vi "FF_AnkleTrajAdv2.vi"(6 "Init":bool, 7 "dt":dbl=0.01 format="%0.2f", 8 "error in (no error)":errorcluster, 9 "AnkleVelocity":dbl[](array[numeric]), 10 "AnkleInGCS":dbl[](array[numeric]), 11 "Force Field Controller in":refnum<class "ForceField.lvclass">) -> (0 "error out":errorcluster, 1 "ClosestPoint":dbl[](array[numeric]), 2 "ForceXYZ":dbl[](array[numeric]), 3 "Force Field Controller out":refnum<class "ForceField.lvclass">, 4 "UpdateTrajPrev":bool, 5 "ForceNTD":dbl[](array[numeric]))   [LabVIEW 2015, in "ForceField.lvclass"]
uses:
  ForceField.lvclass
  ForceField.lvclass/ForceField.ctl
  TypeDef/TND.ctl
  <vilib>/ptbypt/NI_PtbyPt.lvlib
panel:
  out "ToeOffIdx":i32
  in  "3D":bool
  in  "Adv?":bool=TRUE
  out "weightPrev":dbl
  out "ClosePt 2":dbl[](array[numeric])
  in  "HalfWindow 2":i32=35
  in  "dXmin":dbl=0.2 format="%#_13g"
  in  "HalfWindow 1":i32=35
  out "ClosePt 1":dbl[](array[numeric])
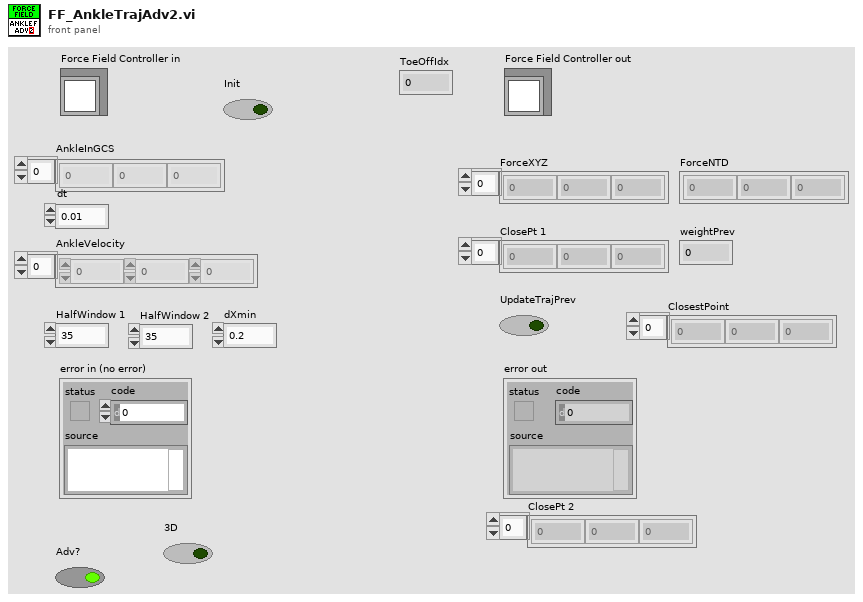
[diagram p1: front panel]
types:
  T1 = typedef "ForceField.lvclass/TND.ctl" = cluster{"Vt":dbl[], "Vn":dbl[], "Dmin":dbl}
  T2 = typedef "ForceField.lvclass/AnkleTrajPt.ctl" = cluster{"P1":dbl[], "P2":dbl[], "P1-P2":dbl[], "(P1-P2)^2":dbl}
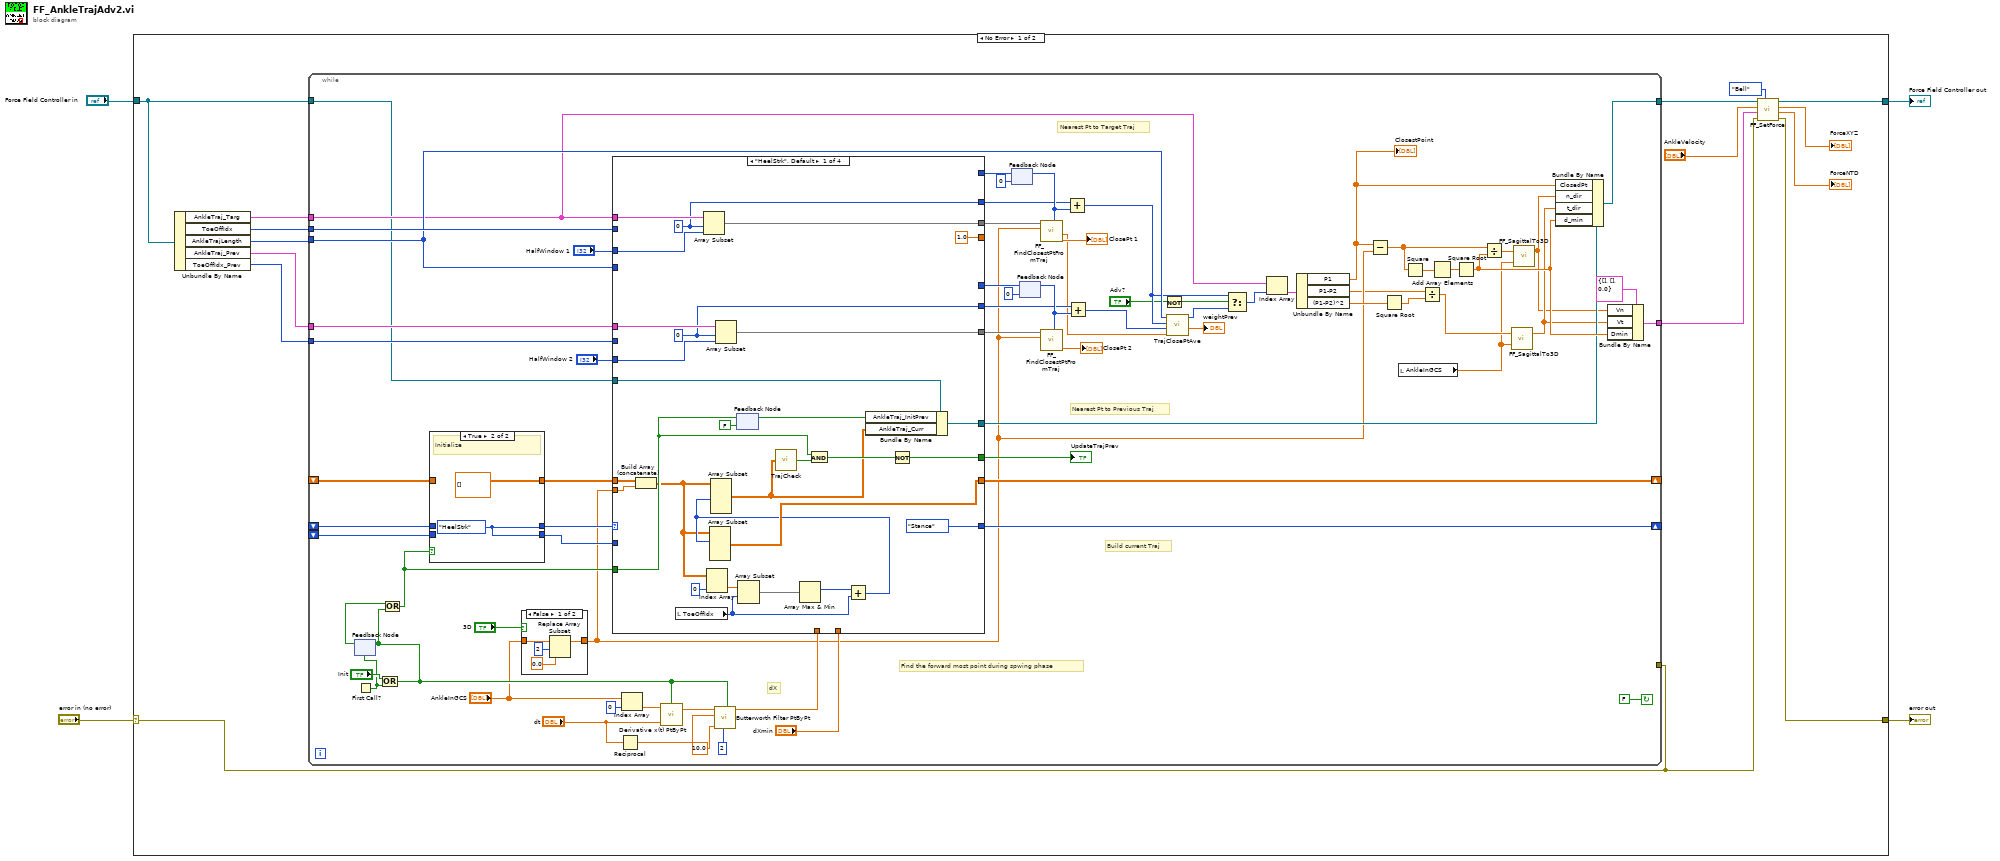
[diagram p0: block diagram]
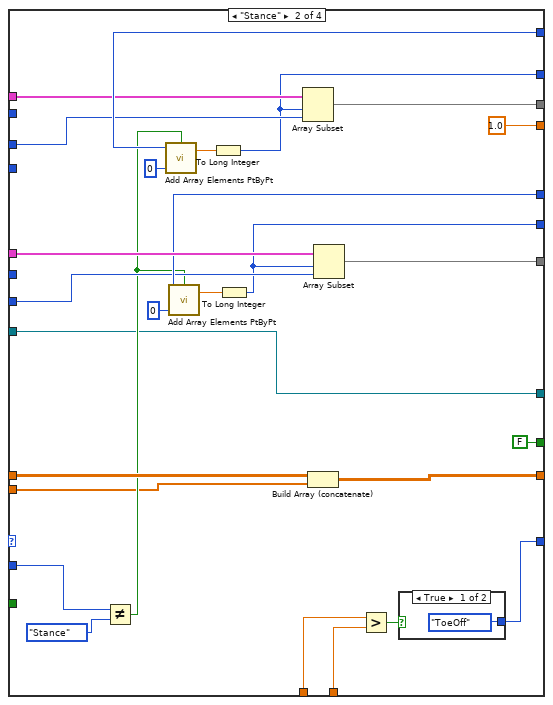
[diagram p3: hidden frame]
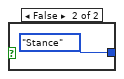
[diagram p4: hidden frame]
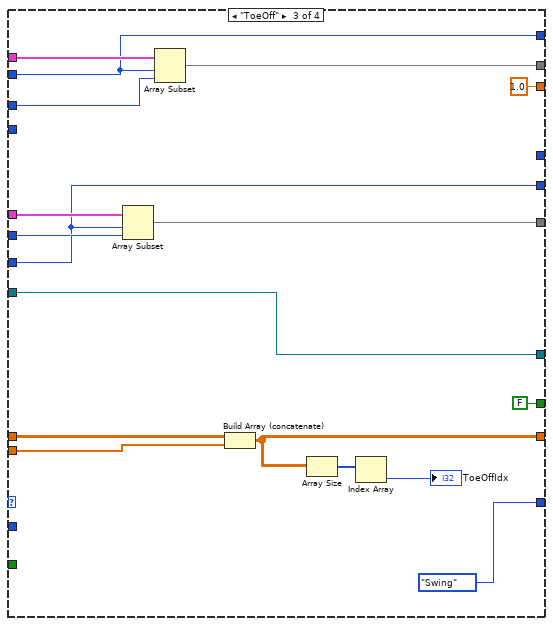
[diagram p5: hidden frame]
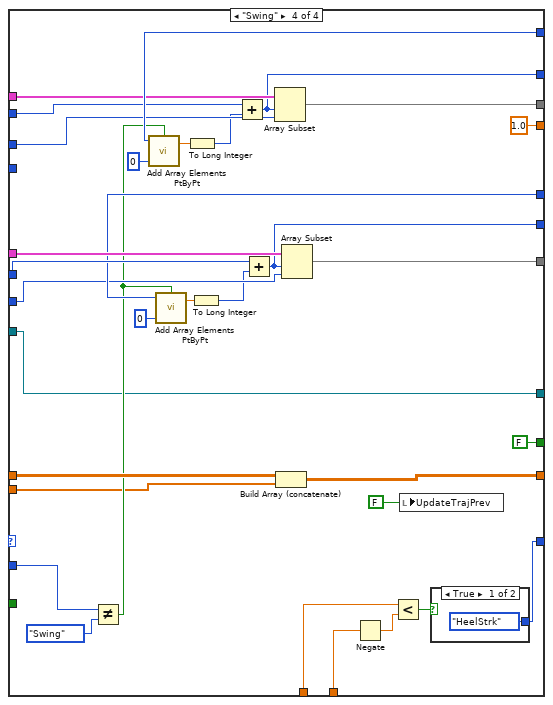
[diagram p6: hidden frame]
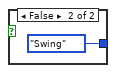
[diagram p7: hidden frame]
diagram:
  n1 = case shown="No Error" "error in (no error)" {
    selector: "error in (no error)" -> [w5 w214]
    tunnel: [w17 w214] -> w3
    tunnel: [w18 w213] -> w1
    tunnel: "Force Field Controller in" -> [w19 w213]
    frame No Error {
      n2 = Unbundle By Name(w19) -> ("AnkleTraj_Targ"=w15:T2[], "ToeOffIdx"=w14:i32, "AnkleTrajLength"=w13:i32, "AnkleTraj_Prev"=w7:T2[], "ToeOffIdx_Prev"=w6:i32)
      n3 = while {
        tunnel: w15 -> [w73]
        tunnel: w14 -> [w84]
        tunnel: w19 -> [w41]
        tunnel: [w92] -> w16
        shift-right: [w87] -> _
        shift-left: _ -> [w79]
        shift-left: _ -> [w77]
        shift-right: [w86] -> _
        shift-left: _ -> [w81]
        tunnel: w13 -> [w82]
        tunnel: w7 -> [w85]
        tunnel: w6 -> [w83]
        tunnel: [w64] -> w12
        tunnel: w5 -> [_]
        stop <- FALSE continue-if-true
        # "dX"
        # "Find the forward most point during spwing phase"
        # "Nearest Pt to Previous Traj"
        # "Build current Traj"
        # "Nearest Pt to Target Traj"
        n4 = First Call?() -> (First Call?: T/F=w74:bool)
        n5 = feedback #1(w74) -> (w75:bool)
        n6 = Or(x="Init", y=w74) -> (x .or. y?=w36:bool)
        n7 = feedback-in #1(w36) -> ()
        n8 = Or(x=w75, y=w36) -> (x .or. y?=w63:bool)
        n9 = case shown="True" w63 {
          tunnel: w81 -> [w210 _]
          tunnel: [w210 dbl[][] []] -> w80
          tunnel: w79 -> [w209 _]
          tunnel: [w209 w211] -> w78
          tunnel: w77 -> [w208 _]
          tunnel: [w208 w211] -> w76
          frame False {
          }
          frame True {
            w211 = enum16{"HeelStrk", "Stance", "ToeOff", "Swing"}."HeelStrk"
            # "Initialize"
          }
        }
        n10 = case shown="False" "3D" {
          tunnel: "AnkleInGCS" -> [w96 w97]
          tunnel: [w95 w97] -> w27
          frame False {
            n11 = Replace Array Subset(array=w96, new element=0.0 ("new element/subarray"), index=2) -> (w95:dbl[])
          }
          frame True {
          }
        }
        n12 = Reciprocal(x="dt") -> (1/x=w34:dbl)
        n13 = Index Array(array="AnkleInGCS", index=0) -> (element=w28:dbl)
        n14 = call <vilib>:"Derivative x(t) PtByPt.vi"("initialize"=w36, "dt"="dt", "x"=w28) -> ("dx/dt"=w38:dbl)  [unwired: 1 in, 1 out]
        n15 = call <vilib>:"Butterworth Filter PtByPt.vi"("initialize"=w36, "order"=2, "low cutoff freq: fl"=10.0, "sampling freq: fs"=w34, "x"=w38) -> ("Filtered x"=w29:dbl)  [unwired: 4 in, 1 out]
        n16 = feedback #2(0 ("IndexOfClosePt")) -> (w61:i32)
        n17 = feedback #3(0 ("IndexOfClosePt")) -> (w55:i32)
        n18 = case shown="\"HeelStrk\", Default" w78 {
          tunnel: w73 -> [w123 w145 w167 w191]
          tunnel: "HalfWindow 1" -> [w124 w152 w170 w204]
          tunnel: [w126 w149 w172 w201] -> w59
          tunnel: [enum16{"HeelStrk", "Stance", "ToeOff", "Swing"}."Stance" w148 enum16{"HeelStrk", "Stance", "ToeOff", "Swing"}."Swing" w199] -> w87
          tunnel: w61 -> [_ w153 _ w205]
          tunnel: w29 -> [_ w147 _ w198]
          tunnel: w76 -> [_ w144 _ w197]
          tunnel: [1.0 1.0 1.0 1.0] -> _
          tunnel: "dXmin" -> [_ w142 _ w194]
          tunnel: w27 -> [w112 w128 w160 w174]
          tunnel: [w105 w141 w158 w192] -> w86
          tunnel: w80 -> [w107 w140 w168 w193]
          tunnel: w82 -> [_ _ _ _]
          tunnel: w85 -> [w121 w138 w166 w186]
          tunnel: "HalfWindow 2" -> [w120 w135 w164 w183]
          tunnel: [w119 w136 w165 w182] -> w54
          tunnel: w84 -> [_ _ w163 w189]
          tunnel: w55 -> [_ w137 _ w184]
          tunnel: w83 -> [_ _ w162 w185]
          tunnel: [w117 w130 w162 w180] -> w51
          tunnel: [w118 w131 w163 w179] -> w49
          tunnel: w63 -> [w108 _ _ _]
          tunnel: w41 -> [w115 w129 w161 w175]
          tunnel: [w113 w129 w161 w175] -> w40
          tunnel: [w110 FALSE FALSE FALSE] -> w30
          frame "HeelStrk", Default {
            w117 = 0 ("index")
            w118 = 0 ("index")
            n19 = Build Array (concatenate)(w107, w112) -> (w103:dbl[][])
            n20 = local read "ToeOffIdx"() -> (w99:i32)
            n21 = Array Subset(array=w123, index=w118, length=w124) -> (w126:T2[])
            n22 = Index Array(array=w103, index (col)=0 ("disabled index (col)")) -> (element=w101:dbl[])  [unwired: 1 in]
            n23 = Array Subset(array=w121, index=w117, length=w120) -> (w119:T2[])
            n24 = feedback-in #4(w108) -> ()
            n25 = feedback #4(FALSE) -> (w114:bool)
            n26 = Array Subset(array=w101, index=w99) -> (w100:dbl[])  [unwired: 1 in]
            n27 = Array Max & Min(array=w100) -> (max index (indices)=w98:i32)  [unwired: 3 out]
            n28 = Add(x=w98, y=w99) -> (x+y=w104:i32)
            n29 = Array Subset(array=w103, index (row)=w104) -> (w105:dbl[][])  [unwired: 3 in]
            n30 = Array Subset(array=w103, length (row)=w104) -> (w106:dbl[][])  [unwired: 3 in]
            n31 = call "TrajCheck.vi"("TrajIn"=w106) -> ("GoodTrajectory?"=w109:bool)
            n32 = And(x=w108, y=w109) -> (x .and. y?=w111:bool)
            n33 = Bundle By Name(cluster=w115, "AnkleTraj_InitPrev"=w114, "AnkleTraj_Curr"=w106) -> (w113:refnum<class "ForceField.lvclass">)
            n34 = Not(x=w111) -> (.not. x?=w110:bool)
          }
          frame "Stance" {
            n35 = Not Equal?(x=w144, y=enum16{"HeelStrk", "Stance", "ToeOff", "Swing"}."Stance") -> (x != y?=w134:bool)
            n36 = call <vilib>:"Add Array Elements PtByPt.vi"("initialize"=w134, "sample length"=0, "input data point"=w153) -> ("sum"=w133:dbl)  [unwired: 1 in, 1 out]
            n37 = call <vilib>:"Add Array Elements PtByPt.vi"("initialize"=w134, "sample length"=0, "input data point"=w137) -> ("sum"=w132:dbl)  [unwired: 1 in, 1 out]
            n38 = To Long Integer(number=w133) -> (32bit integer=w131:i32)
            n39 = To Long Integer(number=w132) -> (32bit integer=w130:i32)
            n40 = Array Subset(array=w145, index=w131, length=w152) -> (w149:T2[])
            n41 = Build Array (concatenate)(w140, w128) -> (w141:dbl[][])
            n42 = Array Subset(array=w138, index=w130, length=w135) -> (w136:T2[])
            n43 = Greater?(x=w147, y=w142) -> (0:w146:bool)
            n44 = case shown="True" w146 {
              tunnel: [enum16{"HeelStrk", "Stance", "ToeOff", "Swing"}."ToeOff" enum16{"HeelStrk", "Stance", "ToeOff", "Swing"}."Stance"] -> w148
              frame True {
              }
              frame False {
              }
            }
          }
          frame "ToeOff" {
            n45 = Array Subset(array=w166, index=w162, length=w164) -> (w165:T2[])
            n46 = Array Subset(array=w167, index=w163, length=w170) -> (w172:T2[])
            n47 = Build Array (concatenate)(w168, w160) -> (w158:dbl[][])
            n48 = Array Size(array=w158) -> (size(s)=w157:i32[])
            n49 = Index Array(array=w157) -> (element=→"ToeOffIdx":i32)  [unwired: 1 in]
          }
          frame "Swing" {
            n50 = Not Equal?(x=w197, y=enum16{"HeelStrk", "Stance", "ToeOff", "Swing"}."Swing") -> (x != y?=w181:bool)
            n51 = call <vilib>:"Add Array Elements PtByPt.vi"("initialize"=w181, "sample length"=0, "input data point"=w205) -> ("sum"=w190:dbl)  [unwired: 1 in, 1 out]
            n52 = call <vilib>:"Add Array Elements PtByPt.vi"("initialize"=w181, "sample length"=0, "input data point"=w184) -> ("sum"=w188:dbl)  [unwired: 1 in, 1 out]
            n53 = To Long Integer(number=w190) -> (32bit integer=w178:i32)
            n54 = To Long Integer(number=w188) -> (32bit integer=w177:i32)
            n55 = Add(x=w189, y=w178) -> (x+y=w179:i32)
            n56 = Add(x=w185, y=w177) -> (x+y=w180:i32)
            n57 = Array Subset(array=w191, index=w179, length=w204) -> (w201:T2[])
            n58 = Build Array (concatenate)(w193, w174) -> (w192:dbl[][])
            n59 = Array Subset(array=w186, index=w180, length=w183) -> (w182:T2[])
            n60 = Negate(x=w194) -> (-x=w195:dbl)
            n61 = Less?(x=w198, y=w195) -> (x < y?=w200:bool)
            n62 = local write "UpdateTrajPrev"(FALSE ("UpdateTrajPrev")) -> ()
            n63 = case shown="True" w200 {
              tunnel: [enum16{"HeelStrk", "Stance", "ToeOff", "Swing"}."HeelStrk" enum16{"HeelStrk", "Stance", "ToeOff", "Swing"}."Swing"] -> w199
              frame True {
              }
              frame False {
              }
            }
          }
        }
        "UpdateTrajPrev" <- w30
        n64 = call "FF_FindClosestPtFromTraj.vi"("AnkleInGCS"=w27, "AnkleTraj"=w59) -> ("ClosestPt"=→"ClosePt 1":dbl[], "DistanceToClosestPt"=w21:dbl, "IndexOfClosePt"=w50:i32)  [unwired: 5 in, 2 out]
        n65 = feedback-in #2(w50) -> ()
        n66 = call "FF_FindClosestPtFromTraj.vi"("AnkleInGCS"=w27, "AnkleTraj"=w54) -> ("ClosestPt"=→"ClosePt 2":dbl[], "IndexOfClosePt"=w52:i32)  [unwired: 5 in, 3 out]
        n67 = feedback-in #3(w52) -> ()
        n68 = Add(x=w49, y=w50) -> (x+y=w45:i32)
        n69 = Add(x=w51, y=w52) -> (x+y=w48:i32)
        n70 = Not(x="Adv?") -> (.not. x?=w43:bool)
        n71 = call "TrajClosePtAve.vi"("Dmin_Target"=w21, "ClosePtIdx_Prev"=w48, "ClosePtIdx_Target"=w45, "TrajLength"=w82) -> ("weightTarget"=→"weightPrev":dbl, "ClosePtIdx_Ave"=w46:i32)  [unwired: 6 in]
        n72 = Select(t=w45, s=w43, f=w46) -> (s? t:f=w62:i32)
        n73 = Index Array(array=w73, index=w62) -> (element=w72:T2)
        n74 = Unbundle By Name(w72) -> ("P1"=w39:dbl[], "P1-P2"=w20:dbl[], "(P1-P2)^2"=w70:dbl)
        "ClosestPoint" <- w39
        n75 = Subtract(x=w39, y=w27) -> (x-y=w67:dbl[])
        n76 = Square Root(x=w70) -> (sqrt(x)=w71:dbl)
        n77 = local read "AnkleInGCS"() -> (w22:dbl[])
        n78 = Square(x=w67) -> (x^2=w69:dbl[])
        n79 = Divide(x=w20, y=w71) -> (x/y=w26:dbl[])
        n80 = Add Array Elements(numeric array=w69) -> (sum=w68:dbl)
        n81 = Square Root(x=w68) -> (sqrt(x)=w65:dbl)
        n82 = Divide(x=w67, y=w65) -> (x/y=w24:dbl[])
        n83 = call "FF_SagittalTo3D.vi"("AnkleInGCS"=w22, "ForceInXY"=w26) -> ("ForceInXYZ"=w25:dbl[])  [unwired: 1 in]
        n84 = call "FF_SagittalTo3D.vi"("AnkleInGCS"=w22, "ForceInXY"=w24) -> ("ForceInXYZ"=w23:dbl[])  [unwired: 1 in]
        n85 = Bundle By Name(cluster=w40, "ClosedPt"=w39, "n_dir"=w23, "t_dir"=w25, "d_min"=w65) -> (w92:refnum<class "ForceField.lvclass">)
        n86 = Bundle By Name(cluster=T1 {"Vt"=[], "Vn"=[], "Dmin"=0.0} ("TND"), "Vn"=w23, "Vt"=w25, "Dmin"=w65) -> (w64:T1)
      }
      n87 = call "FF_SetForce.vi"("Enum"=enum16{"Linear", "Bell"}."Bell", "error in (no error)"=w5, "TND"=w12, "AnkleVelocity"="AnkleVelocity", "Force Field Controller in"=w16) -> ("error out"=w17:errorcluster, "ForceNTD"=→"ForceNTD":dbl[], "ForceXYZ"=→"ForceXYZ":dbl[], "Force Field Controller out"=w18:refnum<class "ForceField.lvclass">)  [unwired: 3 in]
    }
    frame Error {
    }
  }
  "error out" <- w3
  "Force Field Controller out" <- w1
